vi "跑馬燈.vi"() -> ()   [LabVIEW 2015]
panel:
  in  "OK Button":bool
  in  "跑馬燈速度":i32(slide) scale=0.0..100.0
  in  "輸入字串":string
  in  "on color":u32(colorbox)
  in  "off color":u32(colorbox)
  out "Array":bool[][](array[boolean])
  in  "停止":bool
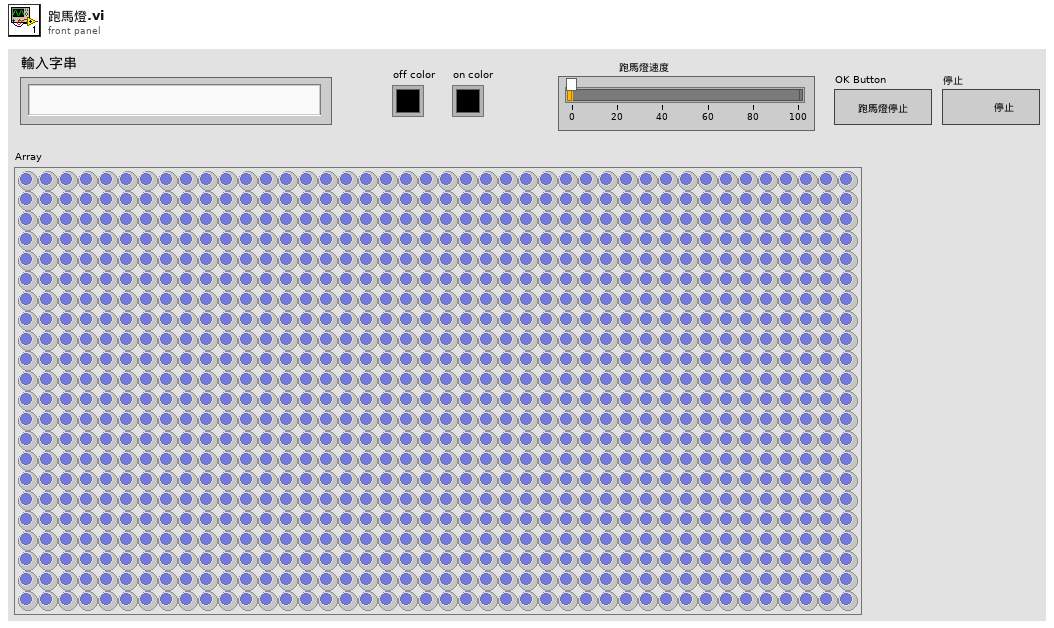
[diagram p1: front panel]
types:
  T1 = cluster{"Font Name:":string, "Size":i16, "Strikeout?":bool, "Italic?":bool, "Underline?":bool, "Outline?":bool, "Shadow?":bool, "Bold?":bool}
  T2 = enum16{"User-specified Font", "Application Font", "System Font", "Dialog Font"}
  T3 = typedef "imagedata.ctl" = cluster{"image type":i32, "image depth":i32, "image":u8[], "mask":u8[], "colors":u32[], "Rectangle":cluster{"left":i16, "top":i16, "right":i16, "bottom":i16}}
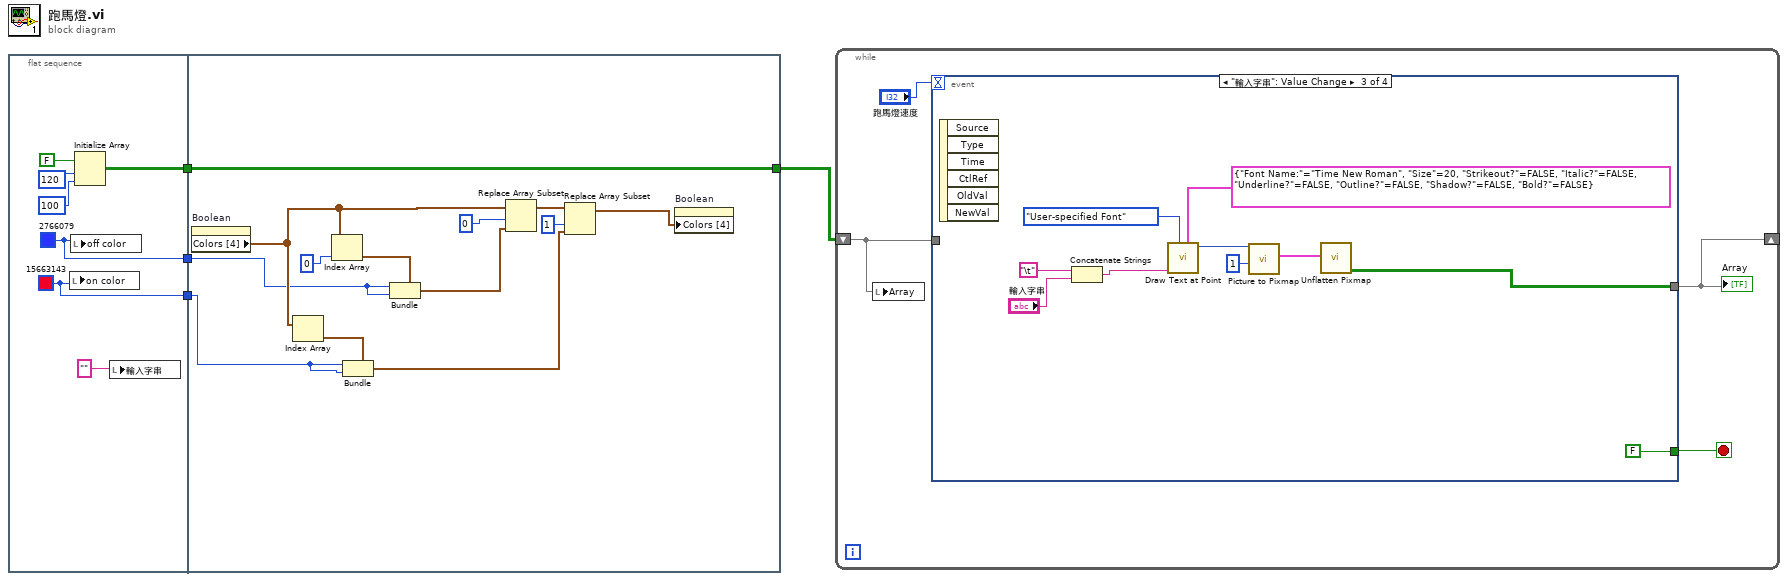
[diagram p0: block diagram]
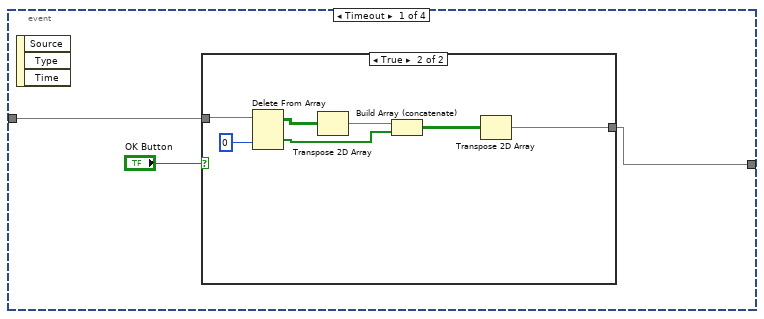
[diagram p2: hidden frame]
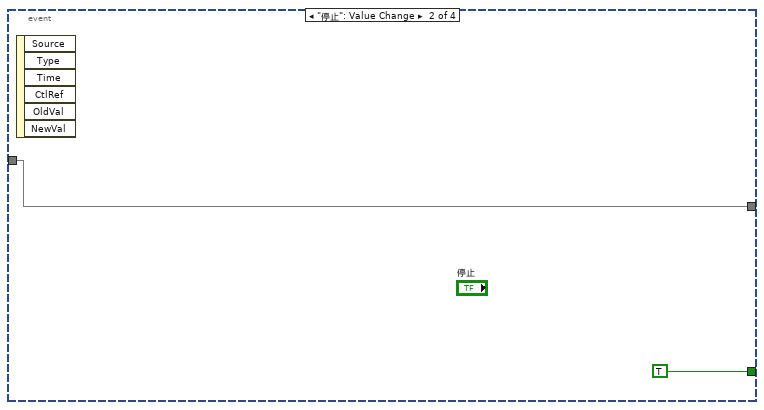
[diagram p4: hidden frame]
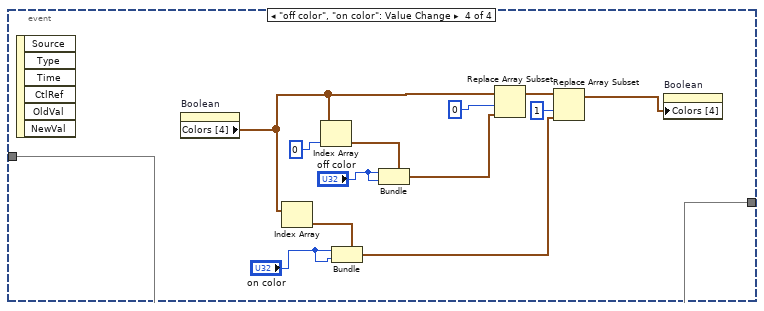
[diagram p5: hidden frame]
diagram:
  n1 = flat-sequence {
    tunnel: [w8] -> w4
    tunnel: [w6] -> w2
    tunnel: [w5] -> w1
    tunnel: w4 -> [w14]
    tunnel: [w14] -> w3
    tunnel: w2 -> [w13]
    tunnel: w1 -> [w12]
    frame #0 {
      w5 = u32 15663143
      w6 = u32 2766079
      n2 = local write "on color"(w5) -> ()
      n3 = local write "off color"(w6) -> ()
      n4 = Initialize Array(FALSE, 120, 100) -> (w8:bool[][])
      n5 = local write "輸入字串"("") -> ()
    }
    frame #1 {
      n6 = property on="Boolean" class="Bool (strict)"() -> ("Colors [4]"=w18:cluster{u32, u32}[])  [unwired: 2 in, 2 out]
      n7 = Index Array(array=w18) -> (element=w16:cluster{u32, u32})  [unwired: 1 in]
      n8 = Index Array(array=w18, index=0) -> (element=w17:cluster{u32, u32})
      n9 = Bundle(cluster=w16, w12, w12) -> (w23:cluster{u32, u32})
      n10 = Bundle(cluster=w17, w13, w13) -> (w20:cluster{u32, u32})
      n11 = Replace Array Subset(array=w18, new element=w20, index=0) -> (w21:cluster{u32, u32}[])
      n12 = Replace Array Subset(array=w21, new element=w23, index=1) -> (w24:cluster{u32, u32}[])
      n13 = property on="Boolean" class="Bool (strict)"("Colors [4]"=w24) -> ()  [unwired: 2 in, 2 out]
    }
  }
  n14 = while {
    shift-right: [w25] -> _
    shift-left: w3 -> [w26]
    stop <- w28 stop-if-true
    n15 = local write "Array"(w26) -> ()
    n16 = event shown="[2] \"輸入字串\": Value Change" {
      selector: _ -> [_ _ _ _]
      dyn-events: _ -> [_ _ _ _]
      timeout: "跑馬燈速度" -> [_ _ _ _]
      tunnel: [_ TRUE FALSE _] -> w28
      tunnel: [w29 w40 w42 w52] -> w25
      tunnel: w26 -> [w30 w40 _ w52]
      event Timeout {
        n17 = event-data() -> ()  [unwired: 1 in, 3 out]
        n18 = case shown="True" "OK Button" {
          tunnel: w30 -> [w32 w39]
          tunnel: [w32 w33] -> w29
          frame False {
          }
          frame True {
            n19 = Delete From Array(array=w39, index (col)=0) -> (deleted portion=w35:bool[], array with subset deleted=w37:bool[][])  [unwired: 2 in]
            n20 = Transpose 2D Array(2D array=w37) -> (transposed array=w36:bool[][])
            n21 = Build Array (concatenate)(w36, w35) -> (w34:bool[][])
            n22 = Transpose 2D Array(2D array=w34) -> (transposed array=w33:bool[][])
          }
        }
      }
      event "停止": Value Change {
        n23 = event-data() -> ()  [unwired: 1 in, 6 out]
      }
      event "輸入字串": Value Change {
        n24 = event-data() -> ()  [unwired: 1 in, 6 out]
        n25 = Concatenate Strings("\t", "輸入字串") -> (w47:string)
        n26 = call <vilib>:"Draw Text at Point.vi"("[user-specified font]"=T1 {"Font Name:"="Time New Roman", "Size"=20, "Strikeout?"=FALSE, "Italic?"=FALSE, "Underline?"=FALSE, "Outline?"=FALSE, "Shadow?"=FALSE, "Bold?"=FALSE}, "desired font(Application)"=T2."User-specified Font", "text"=w47) -> ("new picture"=w45:picture)  [unwired: 7 in, 1 out]
        n27 = call <vilib>:"Picture to Pixmap.vi"("depth"=1, "picture"=w45) -> ("image data"=w43:T3)  [unwired: 8 in, 1 out]
        n28 = call <vilib>:"Unflatten Pixmap.vi"("image data"=w43) -> ("1-bit pixmap"=w42:bool[][])  [unwired: 4 in, 6 out]
      }
      event "off color", "on color": Value Change {
        n29 = event-data() -> ()  [unwired: 1 in, 6 out]
        n30 = property on="Boolean" class="Bool (strict)"() -> ("Colors [4]"=w59:cluster{u32, u32}[])  [unwired: 2 in, 2 out]
        n31 = Index Array(array=w59) -> (element=w63:cluster{u32, u32})  [unwired: 1 in]
        n32 = Index Array(array=w59, index=0) -> (element=w62:cluster{u32, u32})
        n33 = Bundle(cluster=w63, "on color", "on color") -> (w54:cluster{u32, u32})
        n34 = Bundle(cluster=w62, "off color", "off color") -> (w57:cluster{u32, u32})
        n35 = Replace Array Subset(array=w59, new element=w57, index=0) -> (w56:cluster{u32, u32}[])
        n36 = Replace Array Subset(array=w56, new element=w54, index=1) -> (w53:cluster{u32, u32}[])
        n37 = property on="Boolean" class="Bool (strict)"("Colors [4]"=w53) -> ()  [unwired: 2 in, 2 out]
      }
    }
    "Array" <- w25
  }
